vi "test10-LosslessRegisterStatusMultipleTimesNonCSM.vi"(8 "error in (no error)":errorcluster, 11 "TestCase in":refnum<class "testcase-CSMStatusStateRegisterUnregister.lvclass">) -> (0 "error out":errorcluster, 3 "TestCase out":refnum<class "testcase-CSMStatusStateRegisterUnregister.lvclass">)   [LabVIEW 2017, in "testcase-CSMStatusStateRegisterUnregister.lvclass"]
uses:
  testcase-CSMStatusStateRegisterUnregister.lvclass
  <vilib>/addons/_JKI Toolkits/VI Tester/TestCase.llb/TestCase.lvclass
  src/user.lib/_NEVSTOP/Communicable State Machine(CSM)/Communicable State Machine.lvlib
  C:/Program Files (x86)/National Instruments/LabVIEW 2017/vi.lib/addons/_JKI Toolkits/VI Tester/TestCase.llb/TestCase.lvclass
panel:
  out "Arguments":string
  out "ModuleName":string
  out "error out 3":errorcluster
  out "LoopCount":i32
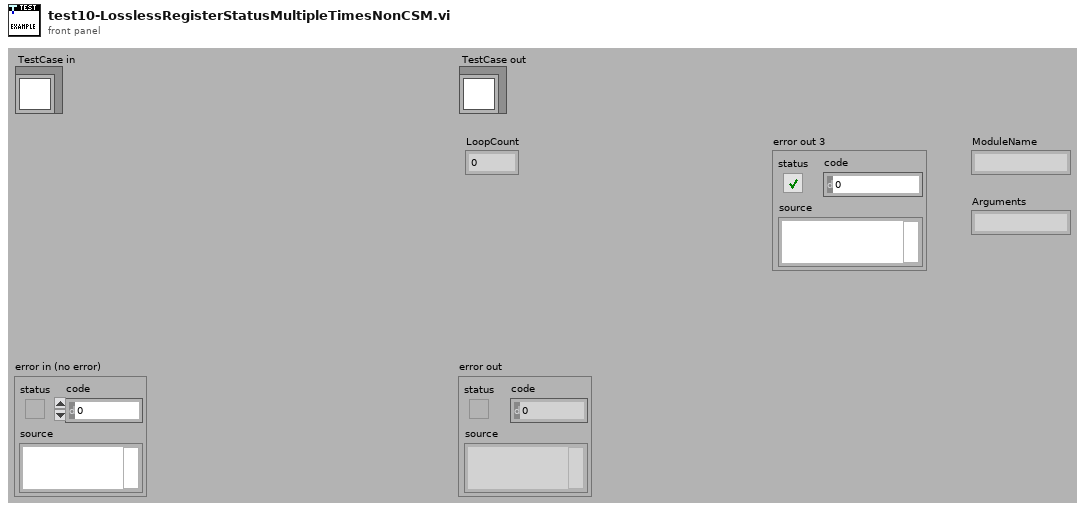
[diagram p1: front panel]
types:
  T1 = cluster{"ModuleName":string, "Status":string, "Arguments":string}
  T2 = cluster{"cluster":cluster{"ModuleName":string, "Status":string, "Arguments":string}, "Counter":u32}
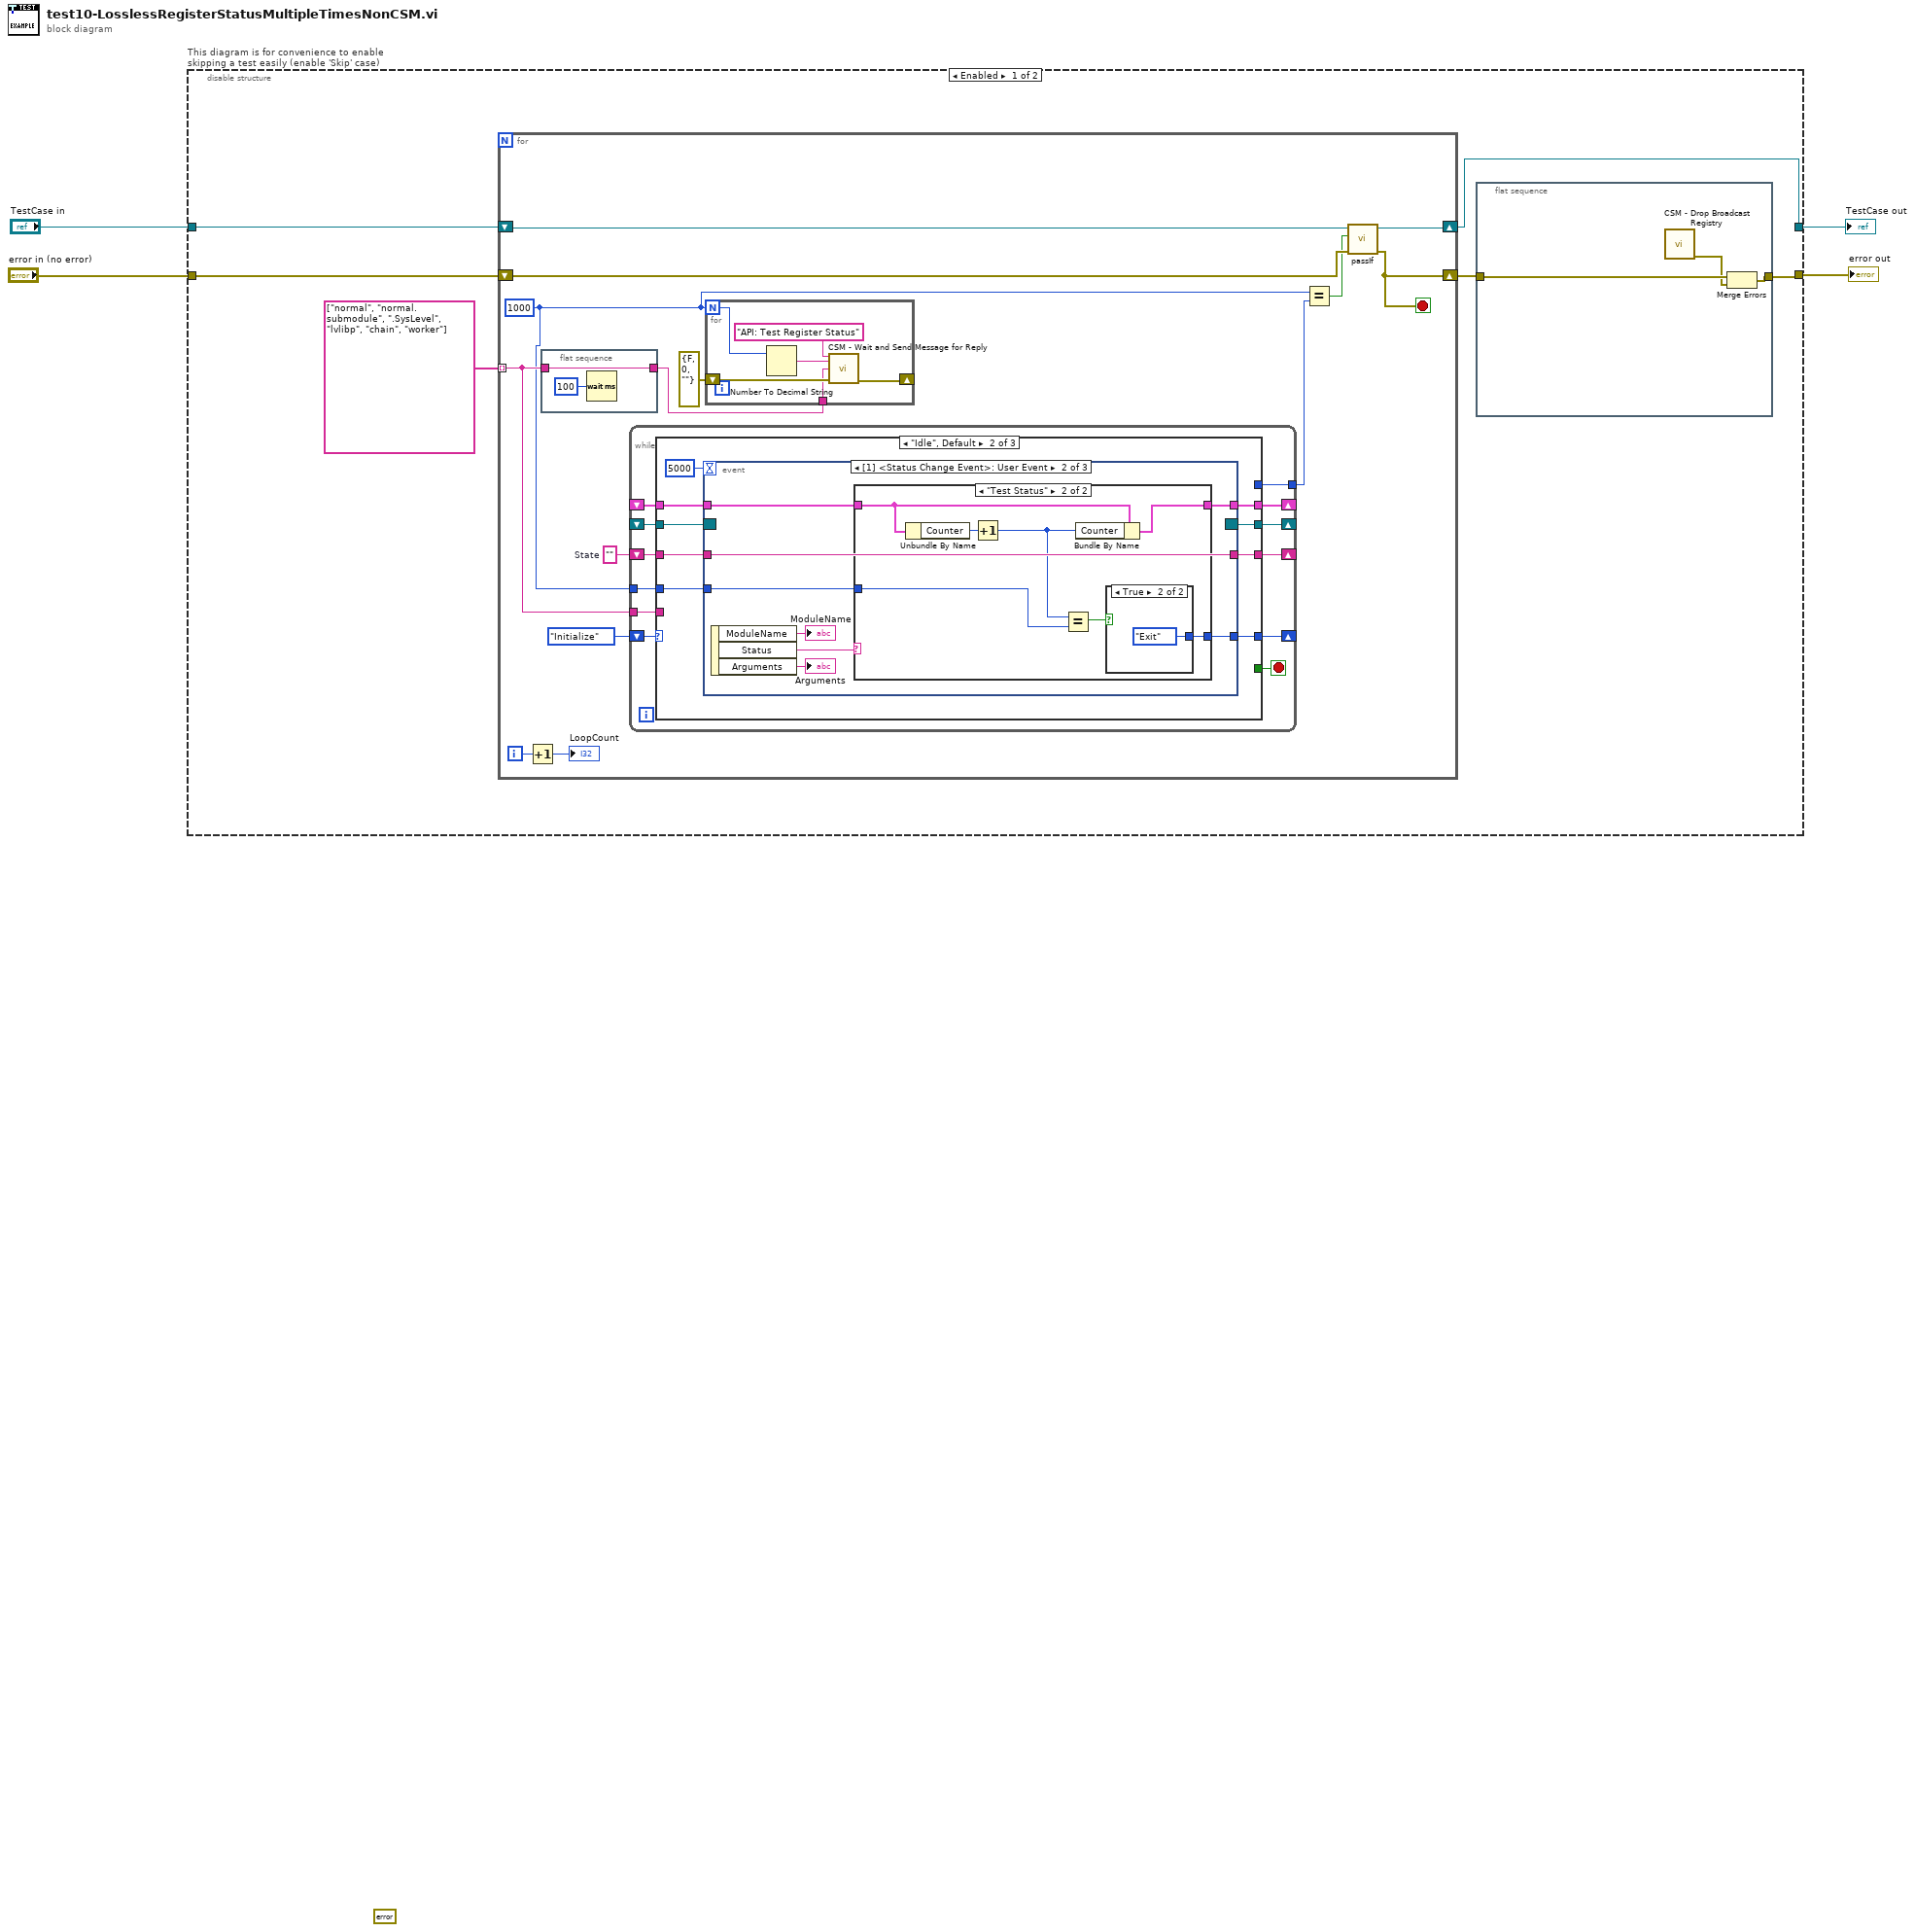
[diagram p0: block diagram]
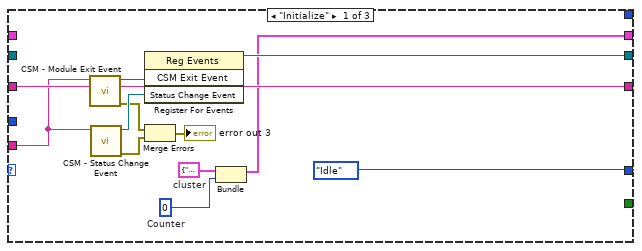
[diagram p2: hidden frame]
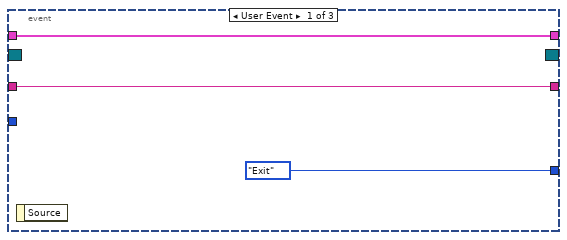
[diagram p3: hidden frame]
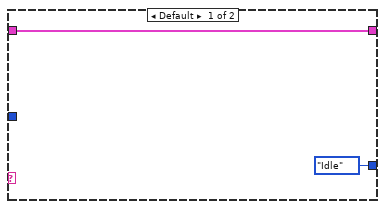
[diagram p4: hidden frame]
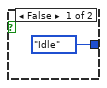
[diagram p5: hidden frame]
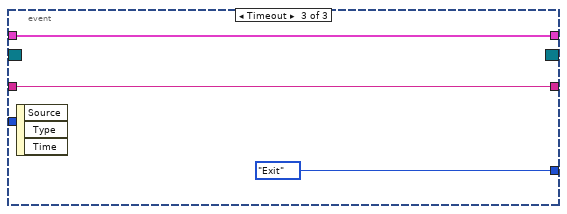
[diagram p6: hidden frame]
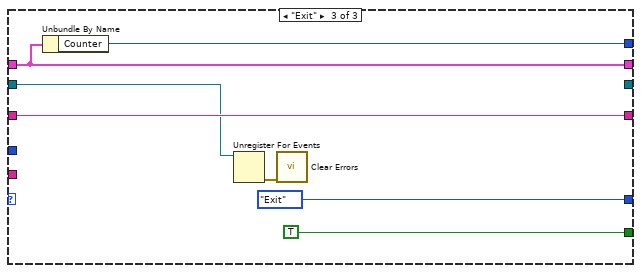
[diagram p7: hidden frame]
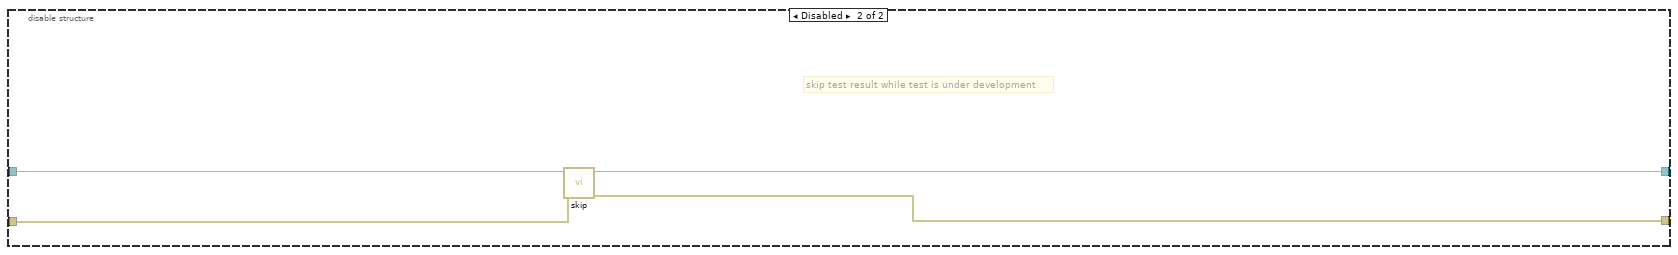
[diagram p8: hidden frame]
diagram:
  (unwired) errorcluster {"status"=FALSE, "code"=0, "source"=""} ("error out")
  n1 = disable-structure "This diagram is for convenience to enable skipping a test easily (enable 'Skip' case)" shown="Enabled" {
    disable-tunnel: "TestCase in" -> [w10 w104]
    disable-tunnel: [w6 w102] -> w2
    disable-tunnel: [w5 w103] -> w1
    disable-tunnel: "error in (no error)" -> [w9 w101]
    frame Enabled {
      n2 = for {
        shift-right: [w24] -> w6
        shift-left: w10 -> [w25]
        shift-right: [w20] -> w7
        shift-left: w9 -> [w23]
        tunnel: string[] ["normal", "normal.submodule", ".SysLevel", "lvlibp", "chain", "worker"] -> [w19] mode=indexing
        i -> [w22]
        stop <- w20 stop-if-true
        w14 = 1000
        w26 = ""  # State
        n3 = Increment(x=w22) -> (x+1=→"LoopCount":i32)
        n4 = flat-sequence {
          tunnel: w19 -> [w35]
          tunnel: [w35] -> w17
          frame #0 {
            n5 = Wait (ms)(milliseconds to wait=u32 100) -> ()  [unwired: 1 out]
          }
        }
        n6 = while {
          shift-right: [w46] -> _
          shift-left: enum16{"Idle", "Initialize", "Exit"}."Initialize" -> [w47]
          shift-right: [w43] -> _
          shift-left: w26 -> [w44]
          shift-right: [w42] -> _
          shift-left: _ -> [w41]
          shift-right: [w40] -> _
          shift-left: _ -> [w39]
          tunnel: w19 -> [w38]
          tunnel: [w37] -> w16
          tunnel: w14 -> [w36]
          stop <- w45 stop-if-true
          n7 = case shown="\"Idle\", Default" w47 {
            tunnel: [enum16{"Idle", "Initialize", "Exit"}."Idle" w68 enum16{"Idle", "Initialize", "Exit"}."Exit"] -> w46
            tunnel: [_ _ TRUE] -> w45
            tunnel: w44 -> [w58 w66 w98]
            tunnel: [w58 w67 w98] -> w43
            tunnel: [w56 w64 _] -> w42
            tunnel: w41 -> [_ w65 w97]
            tunnel: [w55 w62 w94] -> w40
            tunnel: w39 -> [_ w63 w94]
            tunnel: w38 -> [w53 _ _]
            tunnel: [_ _ w95] -> w37
            tunnel: w36 -> [_ w60 _]
            frame "Initialize" {
              w48 = u32 0  # Counter
              w52 = T1 {"ModuleName"="", "Status"="", "Arguments"=""}  # cluster
              n8 = call "CSM - Module Exit Event.vi"("Name (\"\" to Use UUID) In"=w53) -> ("error out"=w51:errorcluster, "CSM Exit Event"=w57:refnum<user-event>)  [unwired: 8 in, 1 out]
              n9 = call "CSM - Status Change Event.vi"("CSM Module"=w53) -> ("error out"=w50:errorcluster, "Status Change Event"=w54:refnum<user-event>)  [unwired: 8 in, 1 out]
              n10 = register-events(w57, w54) -> (reference out=w56:refnum<event-registration>)  [unwired: 2 in, 1 out]
              n11 = Merge Errors(w51, w50) -> (→"error out 3":errorcluster)
              n12 = Bundle("cluster"=w52, "Counter"=w48) -> (w55:T2)  [unwired: 1 in]
            }
            frame "Idle", Default {
              n13 = event shown="[1] <Status Change Event>: User Event" {
                selector: w65 -> [_ _ _]
                dyn-events: [_ _ _] -> w64
                timeout: 5000 -> [_ _ _]
                tunnel: [enum16{"Idle", "Initialize", "Exit"}."Exit" w78 enum16{"Idle", "Initialize", "Exit"}."Exit"] -> w68
                tunnel: w66 -> [w71 w79 w93]
                tunnel: [w71 w79 w93] -> w67
                tunnel: w63 -> [w69 w76 w92]
                tunnel: [w69 w77 w92] -> w62
                tunnel: w60 -> [_ w75 _]
                event User Event {
                  n14 = event-data() -> ()  [unwired: 1 in, 1 out]
                }
                event User Event {
                  n15 = event-data() -> ("ModuleName"=→"ModuleName":string, "Status"=w74:string, "Arguments"=→"Arguments":string)  [unwired: 1 in]
                  n16 = case shown="\"Test Status\"" w74 {
                    tunnel: [enum16{"Idle", "Initialize", "Exit"}."Idle" w88] -> w78
                    tunnel: [w81 w87] -> w77
                    tunnel: w76 -> [w81 w86]
                    tunnel: w75 -> [_ w82]
                    frame Default {
                    }
                    frame "Test Status" {
                      n17 = Unbundle By Name(w86) -> ("Counter"=w85:u32)
                      n18 = Increment(x=w85) -> (x+1=w83:u32)
                      n19 = Equal?(x=w83, y=w82) -> (x = y?=w84:bool)
                      n20 = Bundle By Name(cluster=w86, "Counter"=w83) -> (w87:T2)
                      n21 = case shown="True" w84 {
                        tunnel: [enum16{"Idle", "Initialize", "Exit"}."Idle" enum16{"Idle", "Initialize", "Exit"}."Exit"] -> w88
                        frame False {
                        }
                        frame True {
                        }
                      }
                    }
                  }
                }
                event Timeout {
                  n22 = event-data() -> ()  [unwired: 1 in, 3 out]
                }
              }
            }
            frame "Exit" {
              n23 = Unbundle By Name(w94) -> ("Counter"=w95:u32)
              n24 = Unregister For Events(event registration refnum=w97) -> (error out=w96:errorcluster)  [unwired: 1 in]
              n25 = call <vilib>:"Clear Errors.vi"("error in (no error)"=w96) -> ()  [unwired: 5 in, 2 out]
            }
          }
        }
        n26 = for {
          N: w14 -> [w31]
          shift-right: [w29] -> _
          shift-left: errorcluster {"status"=FALSE, "code"=0, "source"=""} ("error out") -> [w30]
          tunnel: w17 -> [w28]
          n27 = Number To Decimal String(number=w31) -> (decimal integer string=w32:string)  [unwired: 1 in]
          n28 = call "CSM - Wait and Send Message for Reply.vi"("State"="API: Test Register Status", "Arguments (\"\")"=w32, "Target Module"=w28, "Error In (No Error)"=w30) -> ("error out"=w29:errorcluster)  [unwired: 9 in, 2 out]
        }
        n29 = Equal?(x=w14, y=w16) -> (x = y?=w15:bool)
        n30 = call-dynamic "passIf.vi"("error in (no error)"=w23, "pass"=w15, "TestCase in"=w25) -> ("error out"=w20:errorcluster, "TestCase out"=w24:refnum<class "testcase-CSMStatusStateRegisterUnregister.lvclass">)  [unwired: 7 in]
      }
      n31 = flat-sequence {
        tunnel: w7 -> [w13]
        tunnel: [w12] -> w5
        frame #0 {
          n32 = call "CSM - Drop Broadcast Registry.vi"() -> ("error out"=w11:errorcluster)  [unwired: 15 in]
          n33 = Merge Errors(w13, w11) -> (w12:errorcluster)
        }
      }
    }
    frame Disabled {
      # "skip test result while test is under development"
      n34 = call <vilib>:"skip.vi"("error in (no error)"=w101, "TestCase in"=w104) -> ("error out"=w103:errorcluster, "TestCase out"=w102:refnum<class "testcase-CSMStatusStateRegisterUnregister.lvclass">)  [unwired: 8 in]
    }
  }
  "error out" <- w1
  "TestCase out" <- w2
